vi "DictionaryLearning.vi"(8 "error in":errorcluster) -> (0 "error out":errorcluster, 3 "out":refnum<class "DictionaryLearning.lvclass">)   [LabVIEW 2020]
doc: "Dictionary learning\n\n Finds a dictionary (a set of atoms) that can best be used to represent data\n using a sparse code.\n\n Solves the optimization problem::\n\n (U^*,V^*) = argmin 0.5 || X - U V ||_2^2 + alpha * || U ||_1\n (U,V)\n with || V_k ||_2 = 1 for all 0 <= k < n_components\n\n Read more in the :ref:`User Guide <DictionaryLearning>`.\n\n Parameters\n ----------\n n_components : int, default=n_features\n Number of dictionary elements to extract.\n\n alpha : float, default=1.0\n Sparsity controlling parameter.\n\n max_iter : int, default=1000\n Maximum number of iterations to perform.\n\n tol : float, default=1e-8\n Tolerance for numerical error.\n\n fit_algorithm : {'lars', 'cd'}, default='lars'\n * `'lars'`: uses the least angle regression method to solve the lasso\n problem (:func:`~sklearn.linear_model.lars_path`);\n * `'cd'`: uses the coordinate descent method to compute the\n Lasso solution (:class:`~sklearn.linear_model.Lasso`). Lars will be\n faster if the estimated components are sparse.\n\n .. versionadded:: 0.17\n *cd* coordinate descent method to improve speed.\n\n transform_algorithm : {'lasso_lars', 'lasso_cd', 'lars', 'omp', 'threshold'}, default='omp'\n Algorithm used to transform the data:\n\n - `'lars'`: uses the least angle regression method\n (:func:`~sklearn.linear_model.lars_path`);\n - `'lasso_lars'`: uses Lars to compute the Lasso solution.\n - `'lasso_cd'`: uses the coordinate descent method to compute the\n Lasso solution (:class:`~sklearn.linear_model.Lasso`). `'lasso_lars'`\n will be faster if the estimated components are sparse.\n - `'omp'`: uses orthogonal matching pursuit to estimate the sparse\n solution.\n - `'threshold'`: squashes to zero all coefficients less than alpha from\n the projection ``dictionary * X'``.\n\n .. versionadded:: 0.17\n *lasso_cd* coordinate descent method to improve speed.\n\n transform_n_nonzero_coefs : int, default=None\n Number of nonzero coefficients to target in each column of the\n solution. This is only used by `algorithm='lars'` and `algorithm='omp'`\n and is overridden by `alpha` in the `omp` case. If `None`, then\n `transform_n_nonzero_coefs=int(n_features / 10)`.\n\n transform_alpha : float, default=None\n If `algorithm='lasso_lars'` or `algorithm='lasso_cd'`, `alpha` is the\n penalty applied to the L1 norm.\n If `algorithm='threshold'`, `alpha` is the absolute value of the\n threshold below which coefficients will be squashed to zero.\n If `algorithm='omp'`, `alpha` is the tolerance parameter: the value of\n the reconstruction error targeted. In this case, it overrides\n `n_nonzero_coefs`.\n If `None`, default to 1.0\n\n n_jobs : int or None, default=None\n Number of parallel jobs to run.\n ``None`` means 1 unless in a :obj:`joblib.parallel_backend` context.\n ``-1`` means using all processors. See :term:`Glossary <n_jobs>`\n for more details.\n\n code_init : ndarray of shape (n_samples, n_components), default=None\n Initial value for the code, for warm restart. Only used if `code_init`\n and `dict_init` are not None.\n\n dict_init : ndarray of shape (n_components, n_features), default=None\n Initial values for the dictionary, for warm restart. Only used if\n `code_init` and `dict_init` are not None.\n\n verbose : bool, default=False\n To control the verbosity of the procedure.\n\n split_sign : bool, default=False\n Whether to split the sparse feature vector into the concatenation of\n its negative part and its positive part. This can improve the\n performance of downstream classifiers.\n\n random_state : int, RandomState instance or None, default=None\n Used for initializing the dictionary when ``dict_init`` is not\n specified, randomly shuffling the data when ``shuffle`` is set to\n ``True``, and updating the dictionary. Pass an int for reproducible\n results across multiple function calls.\n See :term:`Glossary <random_state>`.\n\n positive_code : bool, default=False\n Whether to enforce positivity when finding the code.\n\n .. versionadded:: 0.20\n\n positive_dict : bool, default=False\n Whether to enforce positivity when finding the dictionary\n\n .. versionadded:: 0.20\n\n transform_max_iter : int, default=1000\n Maximum number of iterations to perform if `algorithm='lasso_cd'` or\n `'lasso_lars'`.\n\n .. versionadded:: 0.22\n\n Attributes\n ----------\n components_ : ndarray of shape (n_components, n_features)\n dictionary atoms extracted from the data\n\n error_ : array\n vector of errors at each iteration\n\n n_iter_ : int\n Number of iterations run.\n\n \nAvailable methods:\nFit\nFit Transform\nTransform\nGet Attributes\nGet Params\nSet Params"
uses:
  DictionaryLearning.lvclass
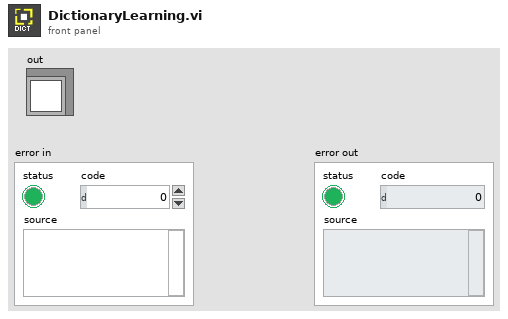
[diagram p1: front panel]
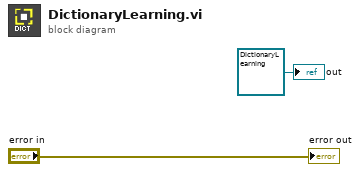
[diagram p0: block diagram]
diagram:
  "out" <- refnum<class "DictionaryLearning.lvclass"> refnum ("model")
  "error out" <- "error in"
